vi "excel_titulos.vi"(4 "input cluster":T1, 5 "error out":errorcluster, 7 "refnum out":refnum<file>) -> (2 "error in":errorcluster, 3 "refnum":refnum<file>)   [LabVIEW 2014]
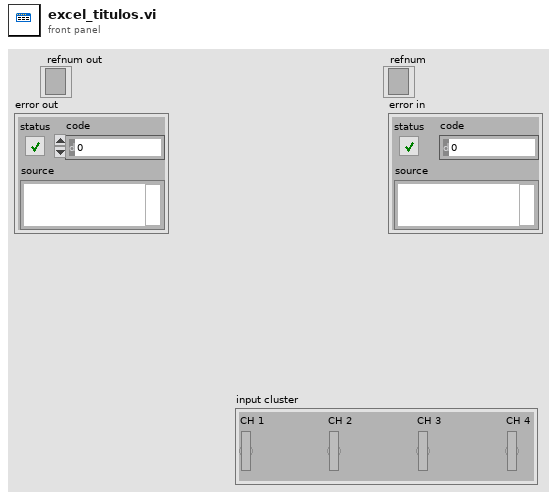
[diagram p1: front panel]
types:
  T1 = cluster{"CH 1":bool, "CH 2":bool, "CH 3":bool, "CH 4":bool}
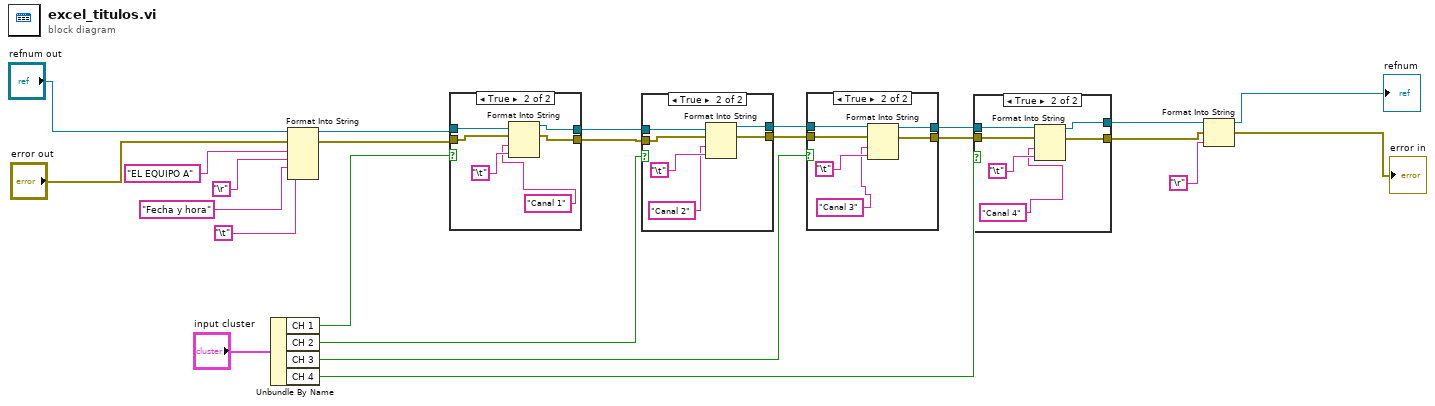
[diagram p0: block diagram]
diagram:
  n1 = Unbundle By Name("input cluster") -> ("CH 1"=w13:bool, "CH 2"=w12:bool, "CH 3"=w11:bool, "CH 4"=w10:bool)
  n2 = Format Into String(initial string="refnum out", error in="error out", "EL EQUIPO A", "\r", "Fecha y hora", "\t") -> (resulting string=w9:refnum<file>, error out=w8:errorcluster)  [unwired: 1 in]
  n3 = case shown="True" w13 {
    tunnel: w9 -> [w26 w32]
    tunnel: w8 -> [w25 w30]
    tunnel: [w26 w31] -> w24
    tunnel: [w25 w29] -> w23
    frame False {
    }
    frame True {
      n4 = Format Into String(initial string=w32, error in=w30, "Canal 1", "\t") -> (resulting string=w31:refnum<file>, error out=w29:errorcluster)  [unwired: 1 in]
    }
  }
  n5 = case shown="True" w12 {
    tunnel: w24 -> [w34 w40]
    tunnel: w23 -> [w33 w37]
    tunnel: [w34 w39] -> w20
    tunnel: [w33 w38] -> w15
    frame False {
    }
    frame True {
      n6 = Format Into String(initial string=w40, error in=w37, "Canal 2", "\t") -> (resulting string=w39:refnum<file>, error out=w38:errorcluster)  [unwired: 1 in]
    }
  }
  n7 = case shown="True" w11 {
    tunnel: w20 -> [w42 w48]
    tunnel: [w42 w47] -> w19
    tunnel: [w41 w46] -> w16
    tunnel: w15 -> [w41 w45]
    frame False {
    }
    frame True {
      n8 = Format Into String(initial string=w48, error in=w45, "Canal 3", "\t") -> (resulting string=w47:refnum<file>, error out=w46:errorcluster)  [unwired: 1 in]
    }
  }
  n9 = case shown="True" w10 {
    tunnel: w19 -> [w50 w56]
    tunnel: [w50 w55] -> w18
    tunnel: [w49 w54] -> w17
    tunnel: w16 -> [w49 w53]
    frame False {
    }
    frame True {
      n10 = Format Into String(initial string=w56, error in=w53, "Canal 4", "\t") -> (resulting string=w55:refnum<file>, error out=w54:errorcluster)  [unwired: 1 in]
    }
  }
  n11 = Format Into String(initial string=w18, error in=w17, "\r") -> (resulting string=→"refnum":refnum<file>, error out=→"error in":errorcluster)  [unwired: 1 in]
